vi "Add Item with Setting.vi"(7 "Tag":string, 8 "error in (no error)":errorcluster, 9 "Setting":T1, 10 "Item":T1, 11 "Application Data in":T2) -> (0 "error out":errorcluster, 2 "new item tag":string, 3 "Application Data out":T2)   [LabVIEW 2020, in "DSF Configuration Utility.lvlib"]
uses:
  DSF Configuration Utility.lvlib
  Tree Item.ctl
  Main VI/Application Data.ctl
  Includes/DSF Core.lvlibp/Classes/Configuration Session/Configuration Session.lvclass
  Main VI/View Mode.ctl
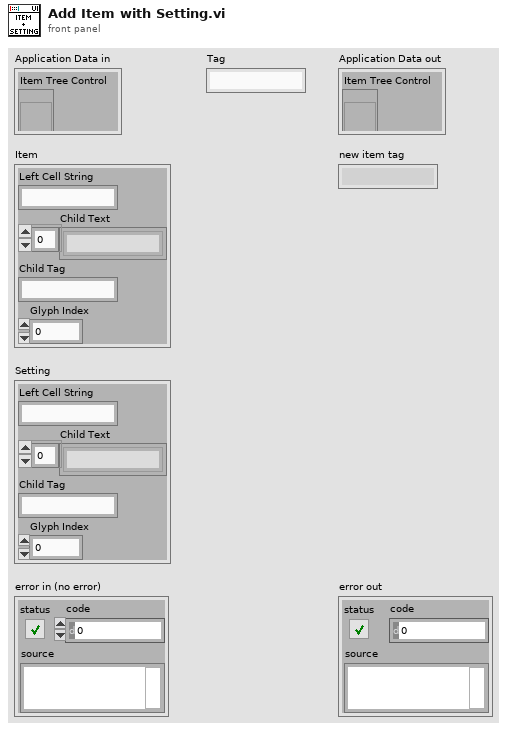
[diagram p1: front panel]
types:
  T1 = typedef "DSF Configuration Utility.lvlib/Tree Item.ctl" = cluster{"Left Cell String":string, "Child Text":string[], "Child Tag":string, "Glyph Index":i32}
  T2 = typedef "DSF Configuration Utility.lvlib/Application Data.ctl" = cluster{"Item Tree Control":refnum<vi>, "Value Tree Control":refnum<vi>, "Configuration Session":refnum<class "Configuration Session.lvclass">, "Top-Level VI":refnum<vi>, "View State":T3, "menu reference":refnum<k9>}
  T3 = typedef "DSF Configuration Utility.lvlib/View Mode.ctl" = enum16{"Tree", "List"}
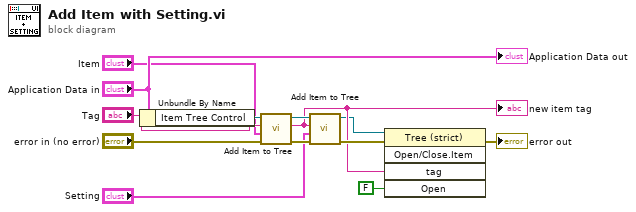
[diagram p0: block diagram]
diagram:
  n1 = Unbundle By Name("Application Data in") -> ("Item Tree Control"=w3:refnum<vi>)
  n2 = call "Add Item to Tree.vi"("error in (no error)"="error in (no error)", "Item"="Item", "parent tag"="Tag", "TreeControl in"=w3) -> ("error out"=w11:errorcluster, "new item tag"=w9:string, "TreeControl out"=w12:refnum<vi>)  [unwired: 5 in]
  "new item tag" <- w9
  n3 = call "Add Item to Tree.vi"("error in (no error)"=w11, "Item"="Setting", "parent tag"=w9, "TreeControl in"=w12) -> ("error out"=w10:errorcluster, "TreeControl out"=w8:refnum<vi>)  [unwired: 5 in, 1 out]
  n4 = invoke class="Tree (strict)" method="Open/Close.Item"(reference=w8, error in=w10, "tag"=w9, "Open"=FALSE ("Open?")) -> (error out=→"error out":errorcluster)  [unwired: 1 in, 4 out]
  "Application Data out" <- "Application Data in"
